vi "Get Multi.vi"(0 "Display State In":T3, 5 "Value In":T1, 9 "Container State":T4, 11 "error in (no error)":errorcluster) -> (4 "Display State Out":T3, 6 "Value Out":T1, 15 "error out":errorcluster)   [LabVIEW 2015, in "Level (G3).xctl"]
uses:
  Level (G3).xctl
  <vilib>/_xctls/Container State.ctl
  State.ctl
  Utility VIs/Controls/KRing/KRing.xctl
  Utility VIs/Controls/KNumeric (DBL)/KNumeric (DBL).xctl
  Level Data.ctl
  Level Units (G3).ctl
  <vilib>/_xctls/XControlSupport.lvlib
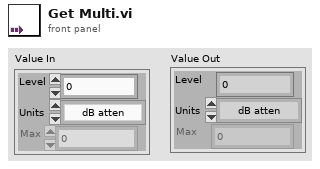
[diagram p1: front panel]
types:
  T1 = typedef "Level (G3).xctl/Level Data.ctl" = cluster{"Level":dbl, "Units":T2, "Max":dbl, "Data":cluster{"Multiplier":dbl, "Cal File":path, "Cal":cluster{"Freq (Hz)":dbl[], "Mag (dB SPL)":dbl[], "Phase (deg)":dbl[]}, "audiogram":path}}
  T2 = typedef "Level (G3).xctl/Level Units (G3).ctl" = enum16{"dB atten", "dB SPL", "dB re 1 Vrms", "dB V/Hz½", "dB SL", "mW", "Volts"}
  T3 = typedef "Level (G3).xctl/State.ctl" = cluster{"LMax Event":refnum<user-event>, "enable menu":bool, "Units":string[], "Valid":bool[], "multi":bool, "ctl":cluster{"Units":refnum<vi>, "Level":refnum<vi>}}
  T4 = typedef "XControlSupport.lvlib/Container State.ctl" = cluster{"Indicator?":bool, "Run Mode?":bool, " Refnum":refnum<vi>}
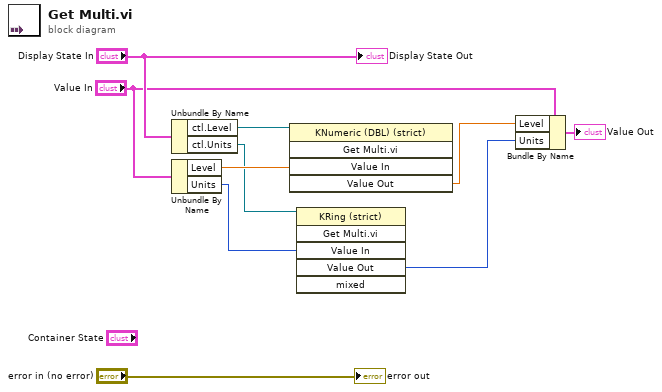
[diagram p0: block diagram]
diagram:
  n1 = Unbundle By Name("Display State In") -> ("ctl.Level"=w8:refnum<vi>, "ctl.Units"=w6:refnum<vi>)
  n2 = Unbundle By Name("Value In") -> ("Level"=w7:dbl, "Units"=w5:T2)
  n3 = invoke class="KNumeric (DBL) (strict)" method="Get Multi.vi"(reference=w8, "Value In"=w7) -> ("Value Out"=w3:dbl)  [unwired: 3 in, 4 out]
  n4 = invoke class="KRing (strict)" method="Get Multi.vi"(reference=w6, "Value In"=w5) -> ("Value Out"=w2:i16)  [unwired: 4 in, 5 out]
  n5 = Bundle By Name(cluster="Value In", "Level"=w3, "Units"=w2) -> (→"Value Out":T1)
  "Display State Out" <- "Display State In"
  "error out" <- "error in (no error)"
